vi "DemoProgram.vi"() -> ()   [LabVIEW 2020]
panel:
  in  "stop":bool
  in  "Boolean":bool
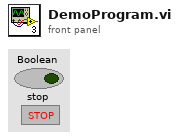
[diagram p1: front panel]
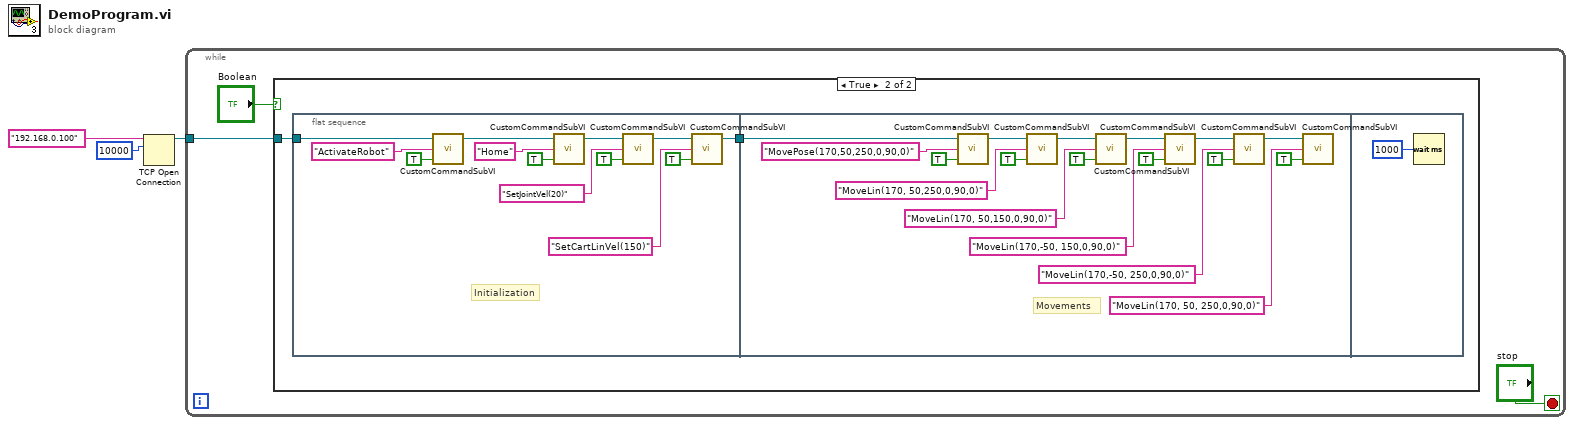
[diagram p0: block diagram]
diagram:
  n1 = TCP Open Connection(address="192.168.0.100", remote port or service name=u16 10000) -> (connection ID=w1:refnum<k5>)  [unwired: 3 in, 1 out]
  n2 = while {
    tunnel: w1 -> [w4]
    stop <- "stop" stop-if-true
    n3 = case shown="True" "Boolean" {
      tunnel: w4 -> [_ w7]
      frame False {
      }
      frame True {
        n4 = flat-sequence {
          tunnel: [w12] -> w8
          tunnel: w7 -> [w9]
          tunnel: w8 -> [w39]
          frame #0 {
            # "Initialization"
            n5 = call "CustomCommandSubVI.vi"("Send_command"=TRUE, "Command"="ActivateRobot", "TCP Network Connection in"=w9) -> ("TCP Network Connection out"=w10:refnum<k5>)  [unwired: 2 out]
            n6 = call "CustomCommandSubVI.vi"("Send_command"=TRUE, "Command"="Home", "TCP Network Connection in"=w10) -> ("TCP Network Connection out"=w11:refnum<k5>)  [unwired: 2 out]
            n7 = call "CustomCommandSubVI.vi"("Send_command"=TRUE, "Command"="SetJointVel(20)", "TCP Network Connection in"=w11) -> ("TCP Network Connection out"=w17:refnum<k5>)  [unwired: 2 out]
            n8 = call "CustomCommandSubVI.vi"("Send_command"=TRUE, "Command"="SetCartLinVel(150)", "TCP Network Connection in"=w17) -> ("TCP Network Connection out"=w12:refnum<k5>)  [unwired: 2 out]
          }
          frame #1 {
            # "Movements"
            n9 = call "CustomCommandSubVI.vi"("Send_command"=TRUE, "Command"="MovePose(170,50,250,0,90,0)", "TCP Network Connection in"=w39) -> ("TCP Network Connection out"=w34:refnum<k5>)  [unwired: 2 out]
            n10 = call "CustomCommandSubVI.vi"("Send_command"=TRUE, "Command"="MoveLin(170, 50,250,0,90,0)", "TCP Network Connection in"=w34) -> ("TCP Network Connection out"=w31:refnum<k5>)  [unwired: 2 out]
            n11 = call "CustomCommandSubVI.vi"("Send_command"=TRUE, "Command"="MoveLin(170, 50,150,0,90,0)", "TCP Network Connection in"=w31) -> ("TCP Network Connection out"=w28:refnum<k5>)  [unwired: 2 out]
            n12 = call "CustomCommandSubVI.vi"("Send_command"=TRUE, "Command"="MoveLin(170,-50, 150,0,90,0)", "TCP Network Connection in"=w28) -> ("TCP Network Connection out"=w25:refnum<k5>)  [unwired: 2 out]
            n13 = call "CustomCommandSubVI.vi"("Send_command"=TRUE, "Command"="MoveLin(170,-50, 250,0,90,0)", "TCP Network Connection in"=w25) -> ("TCP Network Connection out"=w23:refnum<k5>)  [unwired: 2 out]
            n14 = call "CustomCommandSubVI.vi"("Send_command"=TRUE, "Command"="MoveLin(170, 50, 250,0,90,0)", "TCP Network Connection in"=w23) -> ()  [unwired: 3 out]
          }
          frame #2 {
            n15 = Wait (ms)(milliseconds to wait=u32 1000) -> ()  [unwired: 1 out]
          }
        }
      }
    }
  }
